vi "Merge Input Data.vi"(4 "Plot ID":i32, 9 "3D Plot lvclass in":refnum<class "3D Plot Datatype.lvclass">, 11 "3D Plot lvclass Array in":refnum<class "3D Plot Datatype.lvclass">[](array[class])) -> (3 "3D Plot lvclass Array out":refnum<class "3D Plot Datatype.lvclass">[](array[class]))   [LabVIEW 2020, in "3D Plot Datatype.lvclass"]
uses:
  3D Plot Datatype.lvclass
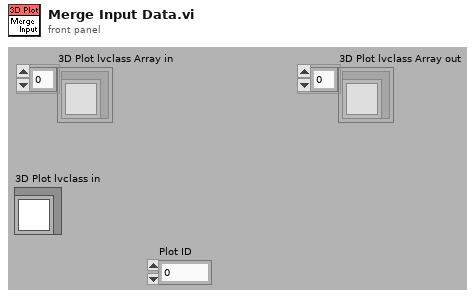
[diagram p1: front panel]
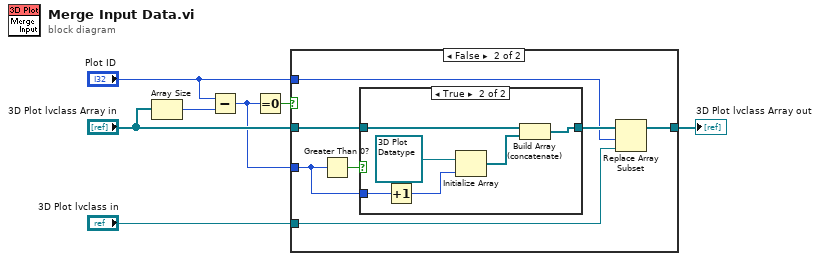
[diagram p0: block diagram]
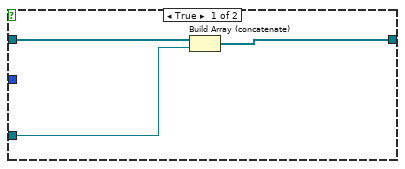
[diagram p2: hidden frame]
diagram:
  n1 = Array Size(array="3D Plot lvclass Array in") -> (size(s)=w7:i32)
  n2 = Subtract(x="Plot ID", y=w7) -> (x-y=w4:i32)
  n3 = Equal To 0?(x=w4) -> (x = 0?=w1:bool)
  n4 = case shown="False" w1 {
    tunnel: "3D Plot lvclass Array in" -> [w10 w16]
    tunnel: w4 -> [_ w11]
    tunnel: [w8 w14] -> w5
    tunnel: "3D Plot lvclass in" -> [w9 w13]
    tunnel: "Plot ID" -> [_ w12]
    frame True {
      n5 = Build Array (concatenate)(w10, w9) -> (w8:refnum<class "3D Plot Datatype.lvclass">[])
    }
    frame False {
      n6 = Greater Than 0?(x=w11) -> (x > 0?=w15:bool)
      n7 = case shown="True" w15 {
        tunnel: w11 -> [_ w23]
        tunnel: [w18 w21] -> w17
        tunnel: w16 -> [w18 w19]
        frame False {
        }
        frame True {
          n8 = Increment(x=w23) -> (x+1=w20:i32)
          n9 = Initialize Array(refnum<class "3D Plot Datatype.lvclass"> refnum ("3D Plot lvclass in 2"), w20) -> (w22:refnum<class "3D Plot Datatype.lvclass">[])
          n10 = Build Array (concatenate)(w19, w22) -> (w21:refnum<class "3D Plot Datatype.lvclass">[])
        }
      }
      n11 = Replace Array Subset(array=w17, new element=w13, index=w12) -> (w14:refnum<class "3D Plot Datatype.lvclass">[])
    }
  }
  "3D Plot lvclass Array out" <- w5
